vi "Timed Loop Mode.vi"() -> ()   [LabVIEW 2023]
doc: "This example illustrates the difference between modes of the Timed Loop that discard pending periods and the modes that process pending periods. One Timed Loop puts an item into a shared queue every 100 ms, while the other loop reads an item every 100 ms (starting with an offset of 1000 ms to wait for the first item to be inserted into the queue). The indicator bars show the number of items sent, received and in the queue at each point.\n\nThe timing of the receiving loop can be controlled by changing the values of the initial delay, a delay introduced in the tenth iteration. Differences between the mode of the receiving loop can be seen by running the VI with different modes."
uses:
  <vilib>/Platform/TimedLoop/XDataNode/nitl_modes.ctl
  <vilib>/Platform/TimedLoop/XDataNode/timing_clust.ctl
  <vilib>/Platform/TimedLoop/XDataNode/wakeup.ctl
  <vilib>/platform/TimedLoop/XDataNode/XDataNode.xnode
  <vilib>/Platform/TimedLoop/XDataNode/XDNodeRunTimeDep.lvlib
panel:
  out "Items Received":i32(slide) scale=0.0..50.0
  out "Items in Queue":i32(slide) scale=0.0..50.0
  out "Items Sent":i32(slide) scale=0.0..50.0
  out "Receiver Finished Late?":bool
  # "Overview: Demonstrates the significance of the Mode configuration value on a Timed Loop.\nRequirements: Windows\nInstructions:\nRun the VI. Observe the number of items sent and received. See the block diagram for more information."
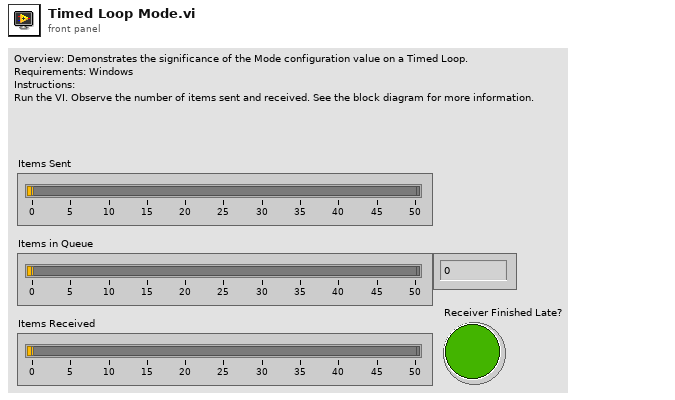
[diagram p1: front panel]
types:
  T1 = typedef "XDNodeRunTimeDep.lvlib/nitl_modes.ctl" = enum32{"No Change", "Process missed periods, maintain original phase", "Discard missed periods, maintain original phase", "Process missed periods, ignore original phase", "Discard missed periods, ignore original phase"}
  T2 = typedef "XDNodeRunTimeDep.lvlib/timing_clust.ctl" = cluster{"Expected End [f-1]":u64, "Actual End [f-1]":u64, "Finished Late? [f-1]":bool, "Expected End [i-1]":u64, "Actual End [i-1]":u64, "Finished Late? [i-1]":bool, "Expected Start [i]":u64, "Actual Start [i]":u64, "Expected Start [f]":u64, "Actual Start [f]":u64, "Source Name":string, "Structure Name":string, "Period":i64, "Deadline":i64, "Offset":i64, "Start":i64, "Priority":i32, "Timeout":i32, "Mode":T1, "Wakeup Reason":T3, "Error":errorcluster, "Source Type":string, "Secondary Source Type":string, "Global End Time":u64, "Global Start Time":u64, "Frame Duration":u64, "Iteration Duration":u64, "Assigned CPU":i32, "I/O Scan Engine Mode":u32}
  T3 = typedef "XDNodeRunTimeDep.lvlib/wakeup.ctl" = enum32{"Normal", "Aborted", "Asynchronous wakeup", "Timing source error", "Timed loop error", "Timeout"}
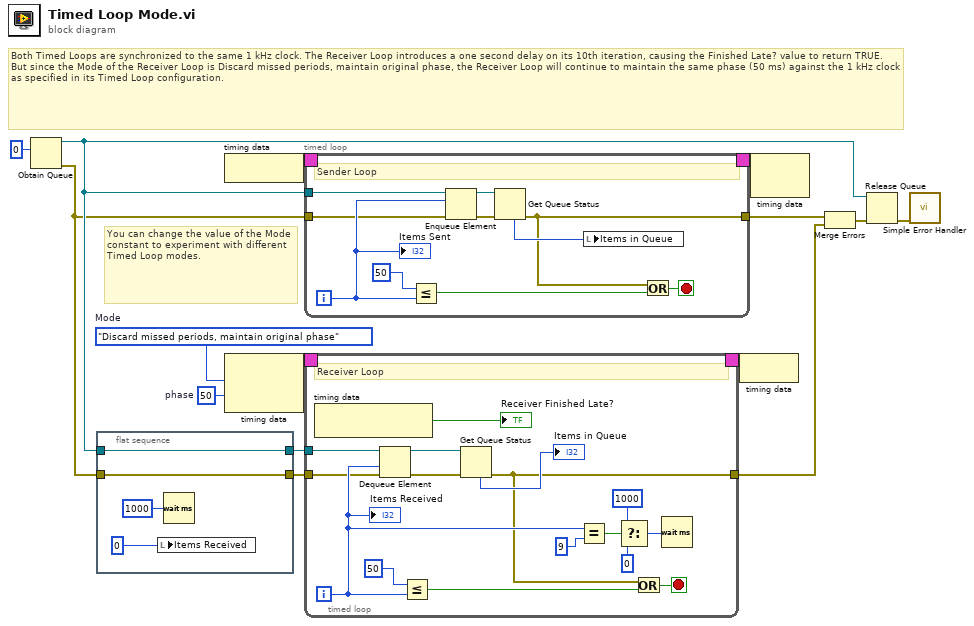
[diagram p0: block diagram]
diagram:
  w1 = i64 50  # phase
  w2 = nitl_modes."Discard missed periods, maintain original phase"  # Mode
  # "You can change the value of the Mode constant to experiment with different Timed Loop modes."
  # "Both Timed Loops are synchronized to the same 1 kHz clock. The Receiver Loop introduces a one second delay on its 10th iteration, causing the Finished Late? value to return TRUE. But since the Mode of the Receiver Loop is Discard missed periods, maintain original phase, the Receiver Loop will continue to maintain the same phase (50 ms) against the 1 kHz clock as specified in its Timed Loop configuration."
  n1 = Obtain Queue(element data type=0) -> (queue out=w10:refnum<queue>, error out=w9:errorcluster)  [unwired: 4 in, 1 out]
  n2 = flat-sequence {
    tunnel: w10 -> [w18]
    tunnel: [w18] -> w4
    tunnel: [w16] -> w3
    tunnel: w9 -> [w16]
    frame #0 {
      n3 = local write "Items Received"(0 ("Items received")) -> ()
      n4 = Wait (ms)(milliseconds to wait=u32 1000 ("Initial \nreceiver delay")) -> ()  [unwired: 1 out]
    }
  }
  n5 = node-c288() -> (w12:T2)
  n6 = node-c288(w2, w1) -> (w7:T2)
  n7 = timed-loop {
    timing: w12 -> [_]
    timing-out: [_] -> w11
    tunnel: w10 -> [w22]
    tunnel: w9 -> [w21]
    tunnel: [w20] -> w8
    i -> [w23]
    stop <- w24 stop-if-true
    # "Sender Loop"
    n8 = Less Or Equal?(x=50, y=w23) -> (x <= y?=w26:bool)
    n9 = Enqueue Element(queue=w22, element=w23, error in (no error)=w21) -> (queue out=w25:refnum<queue>, error out=w28:errorcluster)  [unwired: 1 in, 1 out]
    n10 = Get Queue Status(queue=w25, error in (no error)=w28) -> (error out=w20:errorcluster, # elements in queue=w27:i32)  [unwired: 1 in, 6 out]
    n11 = local write "Items in Queue"(w27) -> ()
    n12 = Or(x=w20, y=w26) -> (x .or. y?=w24:bool)
    "Items Sent" <- w23
  }
  n13 = timed-loop {
    timing: w7 -> [_]
    timing-out: [_] -> w6
    tunnel: [w34] -> w5
    tunnel: w4 -> [w33]
    tunnel: w3 -> [w32]
    i -> [w38]
    stop <- w35 stop-if-true
    # "Receiver Loop"
    n14 = node-c288() -> (→"Receiver Finished Late?":bool)  [unwired: 1 in]
    n15 = Dequeue Element(queue=w33, timeout in ms (-1)=w38, error in (no error)=w32) -> (queue out=w39:refnum<queue>, error out=w47:errorcluster)  [unwired: 2 out]
    n16 = Less Or Equal?(x=50, y=w38) -> (x <= y?=w41:bool)
    n17 = Get Queue Status(queue=w39, error in (no error)=w47) -> (error out=w34:errorcluster, # elements in queue=→"Items in Queue":i32)  [unwired: 1 in, 6 out]
    n18 = Equal?(x=w38, y=9) -> (x = y?=w43:bool)
    n19 = Select(t=u32 1000 ("Receiver delay \nat iteration 10"), s=w43, f=u32 0 ("y")) -> (s? t:f=w44:u32)
    n20 = Or(x=w34, y=w41) -> (x .or. y?=w35:bool)
    n21 = Wait (ms)(milliseconds to wait=w44) -> ()  [unwired: 1 out]
    "Items Received" <- w38
  }
  n22 = node-c288(w6) -> ()
  n23 = node-c288(w11) -> ()  [unwired: 1 out]
  n24 = Merge Errors(w8, w5) -> (w14:errorcluster)
  n25 = Release Queue(queue=w10, error in (no error)=w14) -> (error out=w13:errorcluster)  [unwired: 1 in, 2 out]
  n26 = call <vilib>:"Simple Error Handler.vi"("error in (no error)"=w13) -> ()  [unwired: 4 in, 5 out]
